vi "ExampleInstrument.AppLauncher.vi"() -> ()   [LabVIEW 2016, in "ExampleInstrument.lvclass"]
uses:
  ExampleInstrument.lvclass
  <vilib>/JKI/JKI SMO/SMO/Typedefs/SMOState --Enum.ctl
  Example Instrument UI/ExampleInstrument.UI.lvclass
  C:/Program Files (x86)/National Instruments/LabVIEW 2016/vi.lib/JKI/JKI SMO/SMO/SMO.lvclass
  C:/Program Files (x86)/National Instruments/LabVIEW 2016/vi.lib/JKI/JKI SMO/SMO.UI/SMO.UI.lvclass
  C:/Program Files (x86)/National Instruments/LabVIEW 2016/user.lib/LevyLab/Levylab Instruments/SMOs/Instrument/Instrument.lvclass
  <vilib>/JKI/JKI SMO/SMO/SMO.lvclass
  <vilib>/JKI/JKI SMO/SMO.UI/SMO.UI.lvclass
panel:
  out "error out":errorcluster
  in  "Splash Status":string="Push Start to Start..." caption="String"
  in  "Start":bool=TRUE
  in  "Stop":bool=TRUE
  out "UI SMO State":T1=enum."Stopped"
  out "SMO State":T1
  # "Example Instrument SMO Test Launcher"
  # "For instructions on how to use the JKI State Machine Objects, examples and video tutorials, visit:\nhttp://jki.net/state-machine-objects/\n\nJKI State Machine Objects™\nhttp://jki.net/state-machine-objects/\nCopyright (C) 2005-2015, JKI <info@jki.net>\nALL RIGHTS RESERVED"
  # "Starting Example Instrument..."
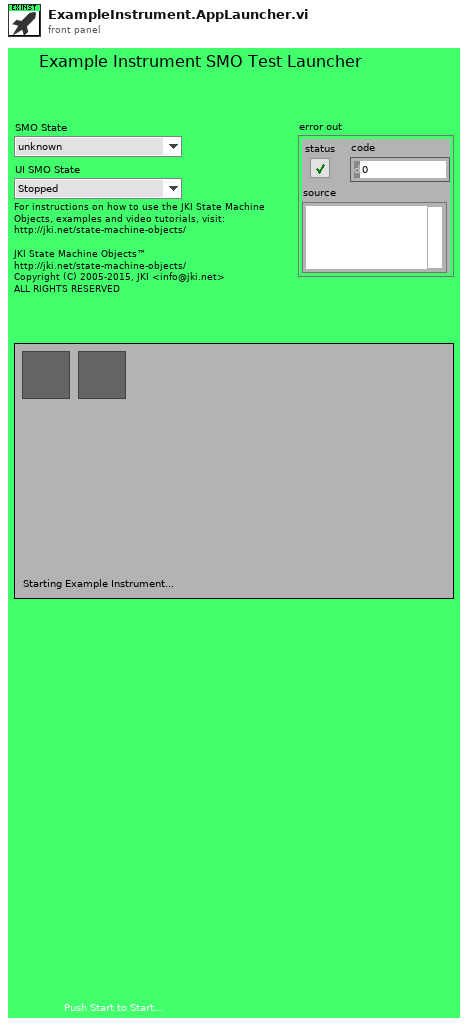
[diagram p1: front panel]
types:
  T1 = typedef "SMO.lvclass/SMOState --Enum.ctl" = enum16{"unknown", "Created", "Started", "Stopped"}
  T2 = enum32{"Invalid", "Standard", "Closed", "Hidden", "Minimized", "Maximized"}
  T3 = enum32{"invalid app kind", "Development System", "Run Time System", "Student Edition", "Embedded LabVIEW", "Evaluation", "Custom"}
  T4 = cluster{"Core":cluster{"Current VI Reference":refnum<vi>, "Close Panel on Exit?":bool}, "Instrument":refnum<class "ExampleInstrument.lvclass">, "Instrument UI":refnum<class "ExampleInstrument.UI.lvclass">}
  T5 = cluster{"Current VI Reference":refnum<vi>, "Close Panel on Exit?":bool}
  T6 = typedef "SMO.lvclass/Public Events.ctl" = cluster{"Error":refnum<user-event>, "State":refnum<user-event>, "Reserve State":refnum<user-event>}
  T7 = cluster{"Event Registration Refnum":refnum<event-registration>, "Event Registration Refnum":refnum<event-registration>}
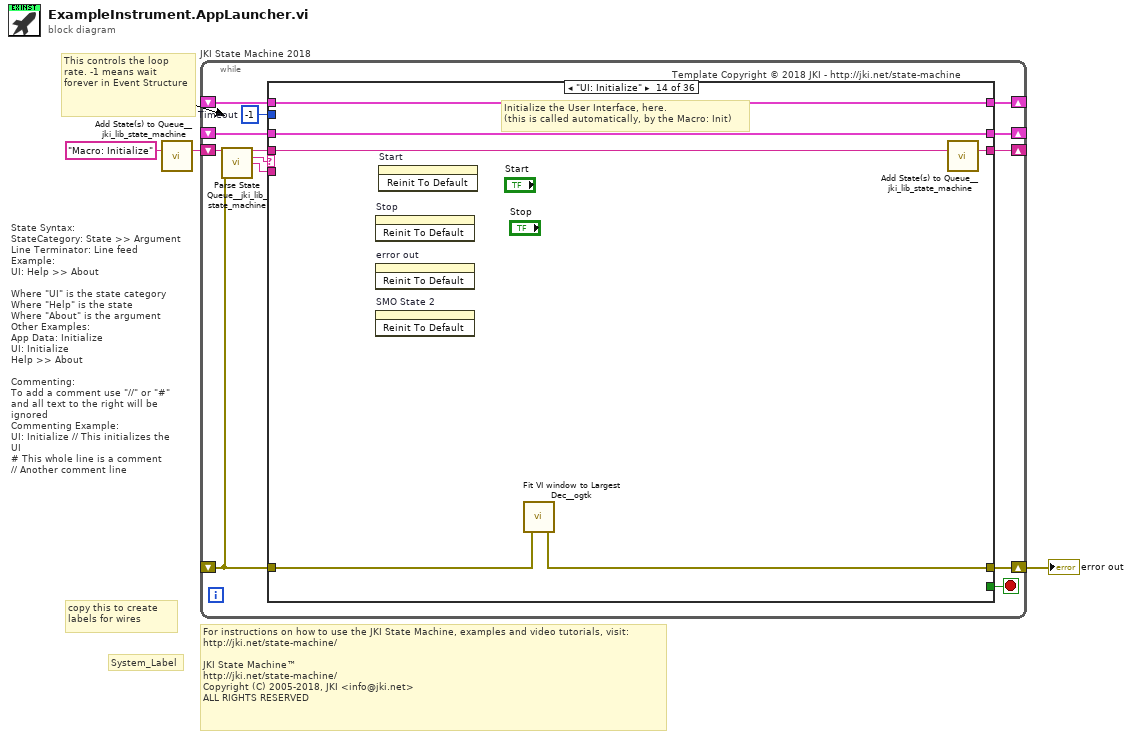
[diagram p0: block diagram]
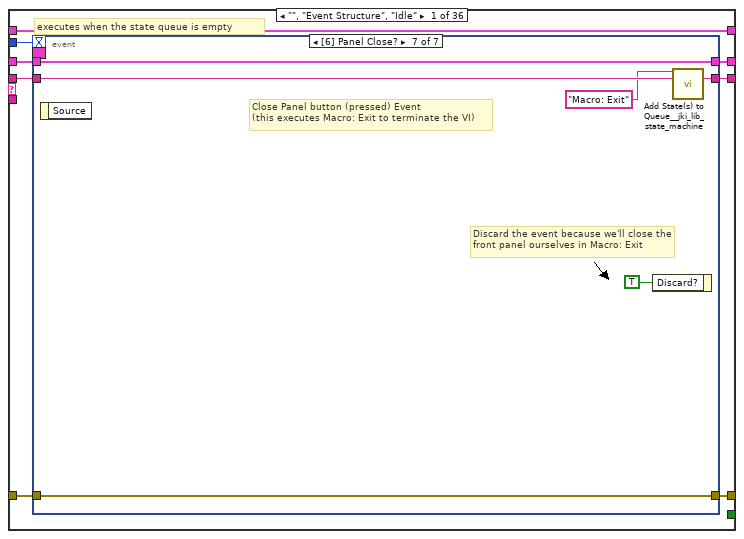
[diagram p2: hidden frame]
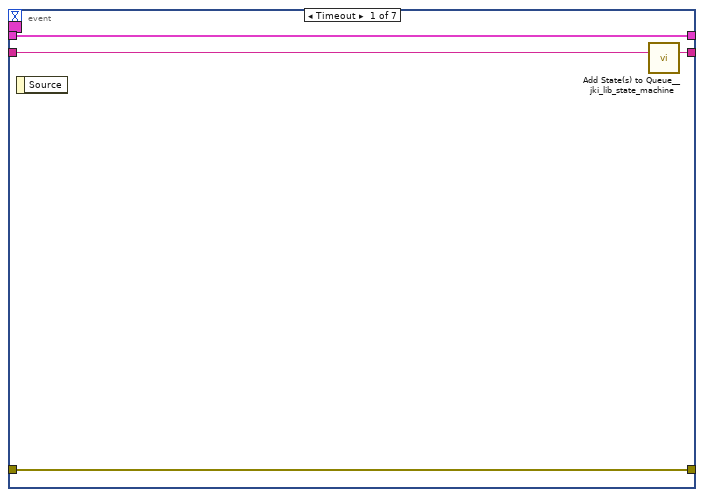
[diagram p3: hidden frame]
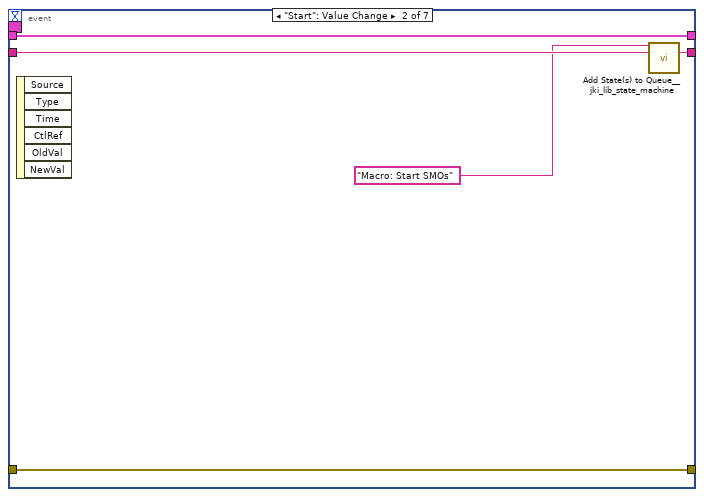
[diagram p4: hidden frame]
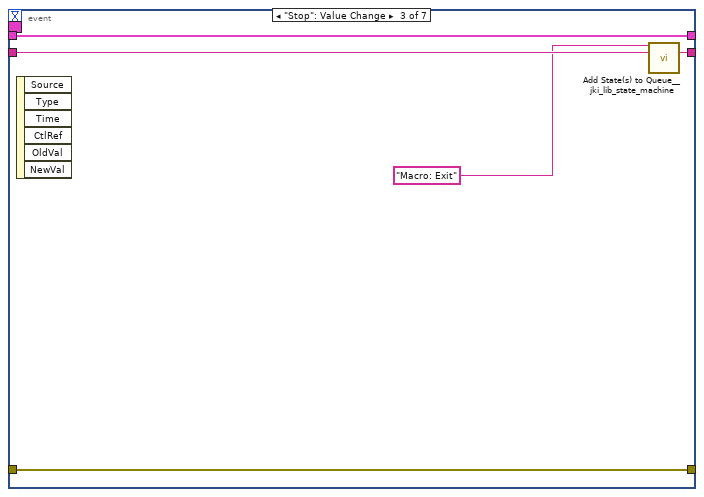
[diagram p5: hidden frame]
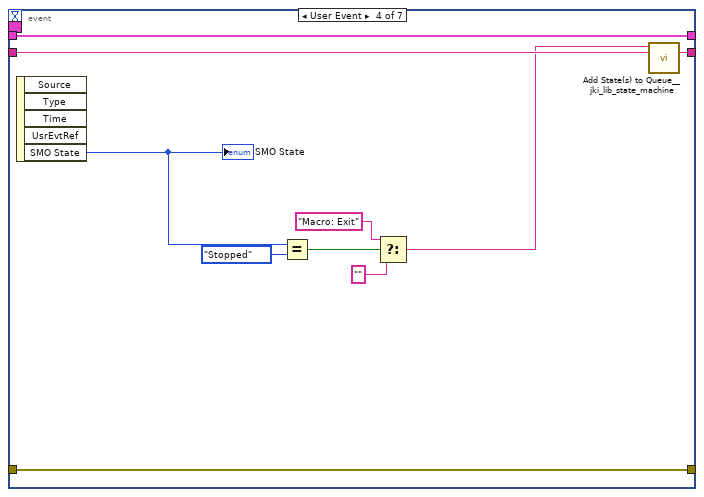
[diagram p6: hidden frame]
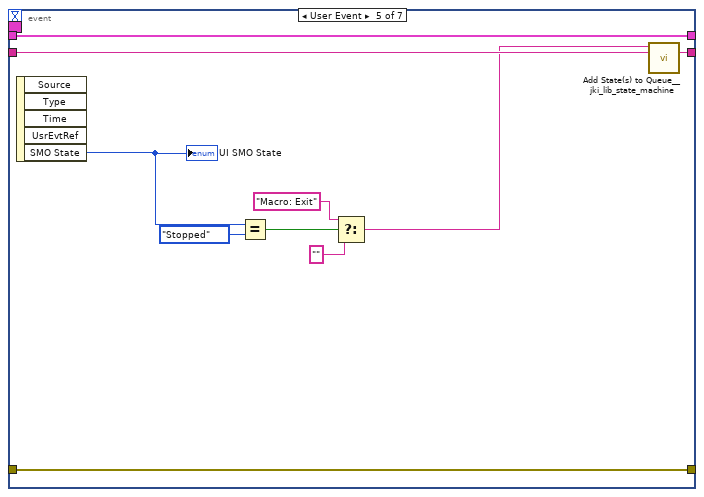
[diagram p7: hidden frame]
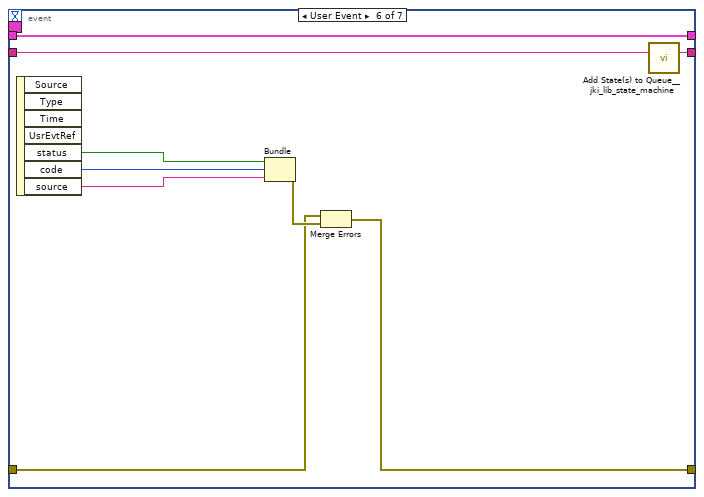
[diagram p8: hidden frame]
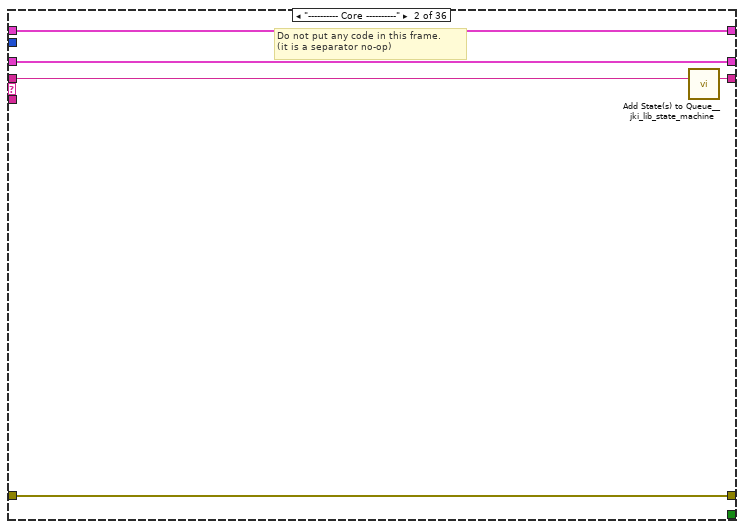
[diagram p9: hidden frame]
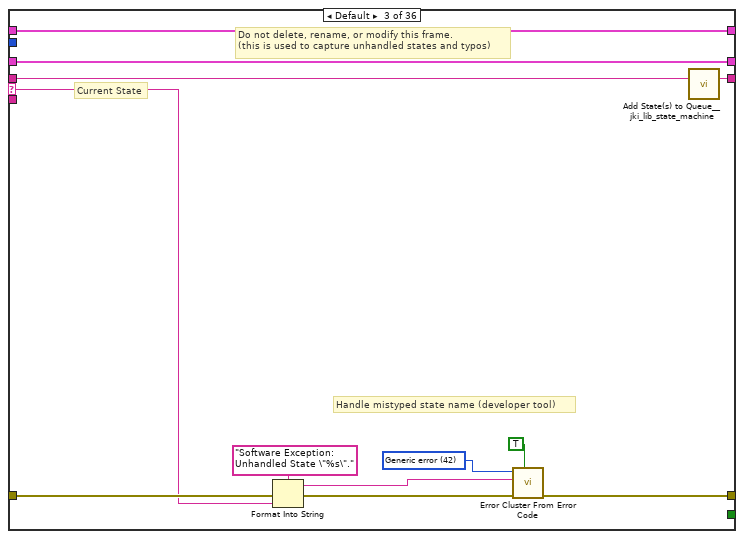
[diagram p10: hidden frame]
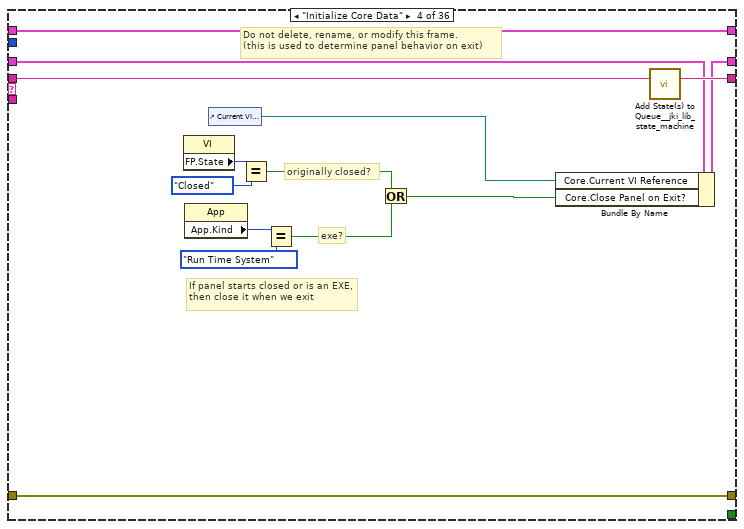
[diagram p11: hidden frame]
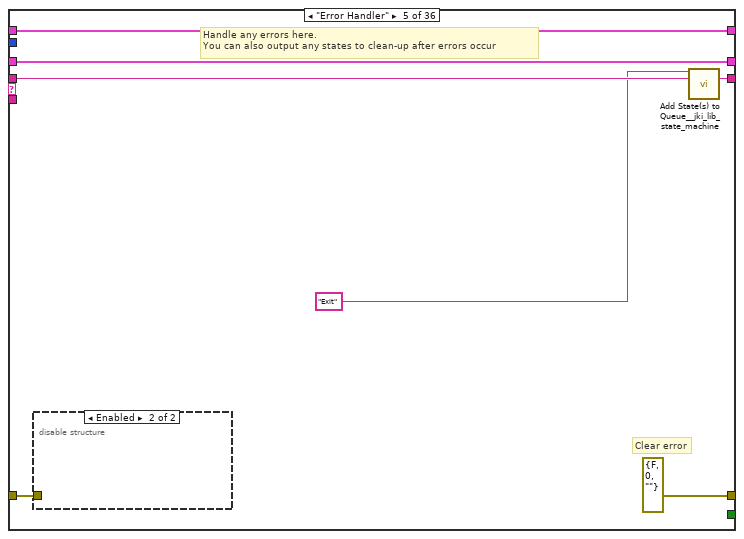
[diagram p12: hidden frame]
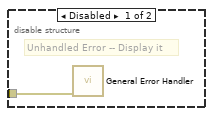
[diagram p13: hidden frame]
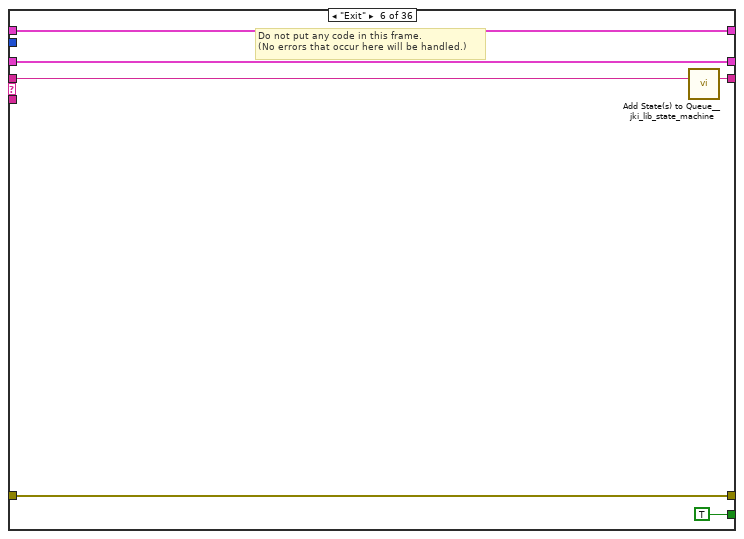
[diagram p14: hidden frame]
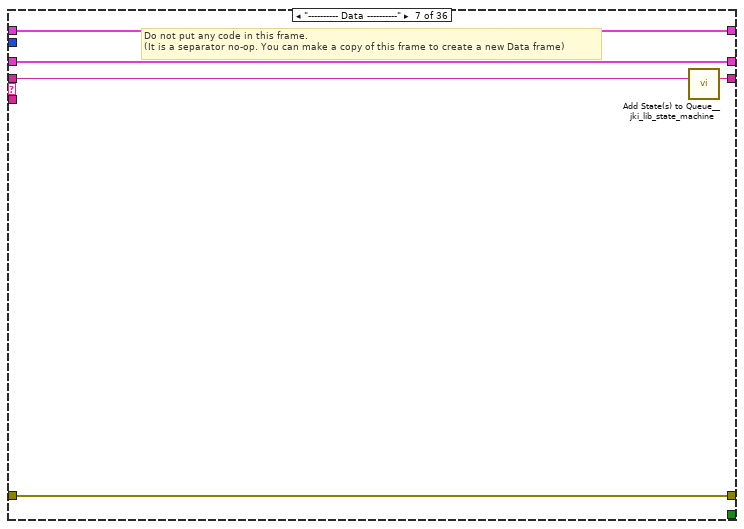
[diagram p15: hidden frame]
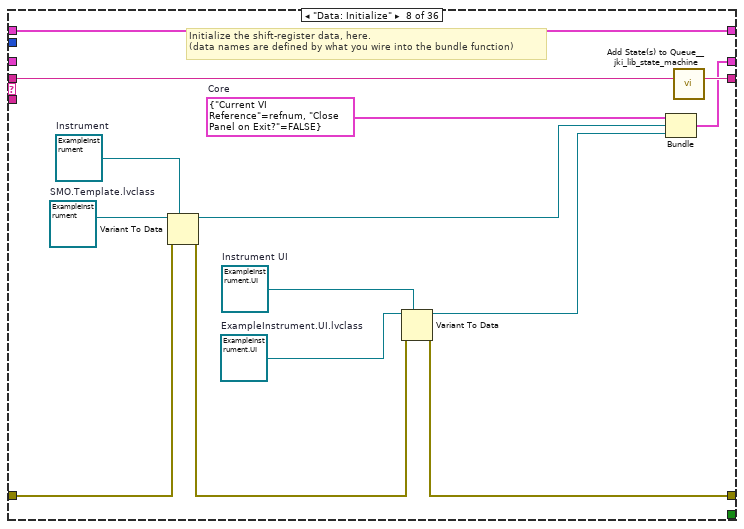
[diagram p16: hidden frame]
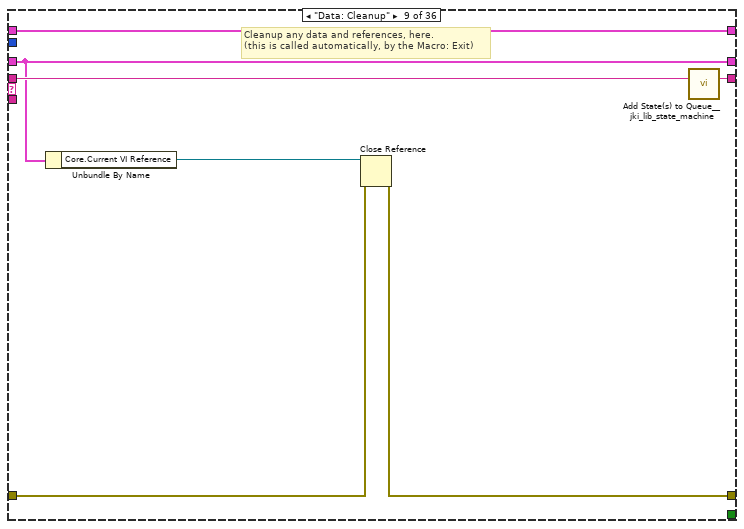
[diagram p17: hidden frame]
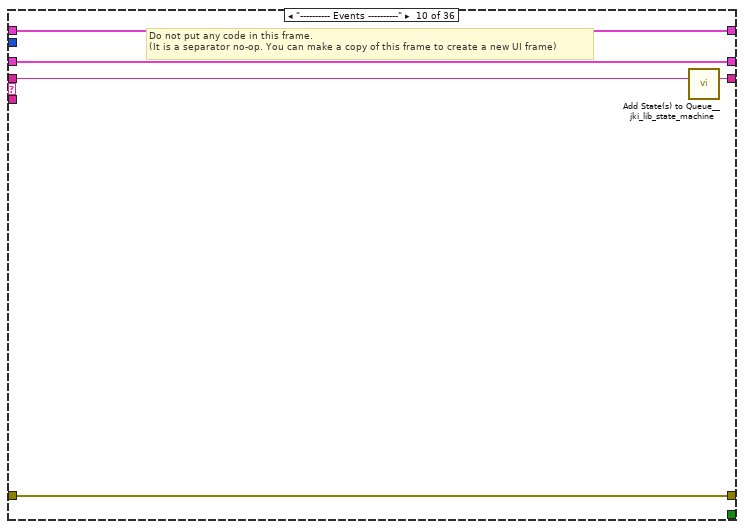
[diagram p18: hidden frame]
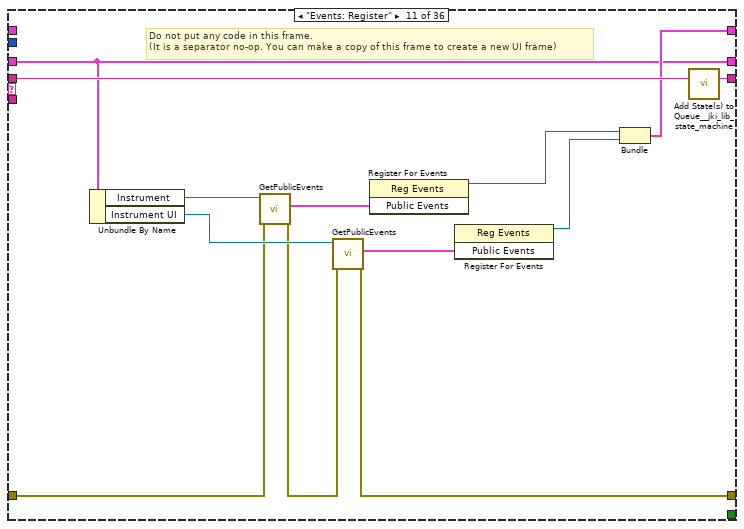
[diagram p19: hidden frame]
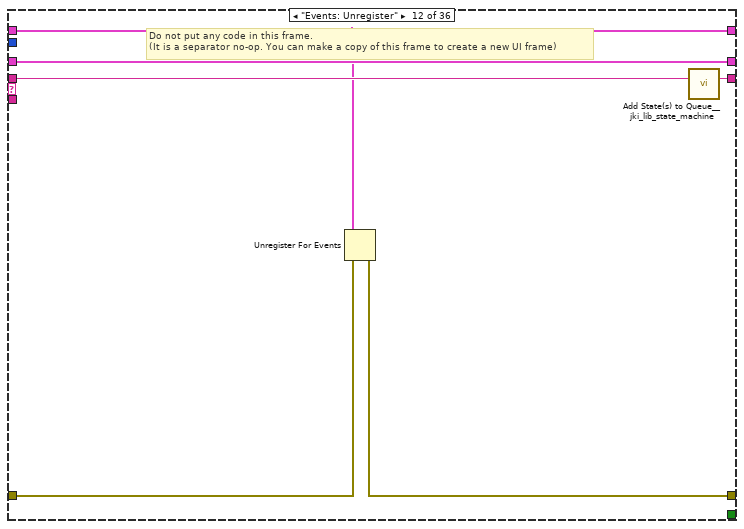
[diagram p20: hidden frame]
diagram:
  # "For instructions on how to use the JKI State Machine, examples and video tutorials, visit:\nhttp://jki.net/state-machine/\n\nJKI State Machine™\nhttp://jki.net/state-machine/\nCopyright (C) 2005-2018, JKI <info@jki.net>\nALL RIGHTS RESERVED"
  # "State Syntax:\nStateCategory: State >> Argument\nLine Terminator: Line feed\nExample:\nUI: Help >> About\n\nWhere \"UI\" is the state category\nWhere \"Help\" is the state\nWhere \"About\" is the argument\nOther Examples:\nApp Data: Initialize\nUI: Initialize\nHelp >> About\n\nCommenting:\nTo add a comment use \"//\" or \"#\" and all text to the right will be ignored\nCommenting Example:\nUI: Initialize // This initializes the UI\n# This whole line is a comment\n// Another comment line"
  # "copy this to create labels for wires"
  # "This controls the loop rate. -1 means wait forever in Event Structure"
  # "System_Label"
  n1 = call <vilib>:"Add State(s) to Queue__jki_lib_state_machine.vi"("State(s) in (\"\")"="Macro: Initialize") -> ("States Out"=w3:string)  [unwired: 14 in]
  n2 = while "JKI State Machine 2018" {
    shift-right: [w9] -> _
    shift-left: _ -> [w4]
    shift-right: [w12] -> w1
    shift-left: _ -> [w7]
    shift-right: [w11] -> _
    shift-left: w3 -> [w13]
    shift-right: [w6] -> _
    shift-left: _ -> [w5]
    stop <- w10 stop-if-true
    w8 = -1  # Timeout
    # "Template Copyright © 2018 JKI - http://jki.net/state-machine"
    n3 = call <vilib>:"Parse State Queue__jki_lib_state_machine.vi"("State Queue"=w13, "Error In (no error)"=w7) -> ("Remaining States"=w15:string, "Current State"=w16:string, "Arguments"=w14:string)  [unwired: 11 in]
    n4 = case shown="\"UI: Initialize\"" w16 {
      selector: w16 -> [_ _ w80 _ _ _ _ _ _ _ _ _ _ _ _ _ _ _ _ _ _ _ _ _ _ _ _ _ _ _ _ _ _ _ _ _]
      tunnel: w15 -> [w24 w78 w84 w104 w111 w118 w123 w137 w144 w149 w162 w168 w173 w179 w186 w198 w276 w281 w286 w292 w298 w304 w316 w321 w330 w339 w349 w356 w367 w382 w397 w412 w427 w436 w443 w448]
      tunnel: w14 -> [_ _ _ _ _ _ _ _ _ _ _ _ _ _ w181 w192 _ _ _ _ _ _ _ _ _ _ _ _ _ _ _ _ _ _ w440 _]
      tunnel: [w21 w76 w86 w101 errorcluster {"status"=FALSE, "code"=0, "source"=""} ("error out") w115 w121 w125 w140 w147 w151 w163 w171 w174 w182 w195 w266 w279 w284 w290 w296 w302 w314 w319 w326 w331 w340 w350 w363 w378 w393 w409 w424 w434 w438 w446] -> w12
      tunnel: w7 -> [w20 w76 w85 w101 w107 w115 w121 w127 w141 w147 w153 w164 w171 w176 w183 w196 w267 w279 w284 w290 w296 w302 w314 w319 w327 w332 w341 w351 w360 w374 w390 w407 w420 w434 w439 w446]
      tunnel: [w23 w77 w83 w103 w110 w117 w122 w136 w143 w148 w161 w167 w172 w178 w185 w197 w275 w280 w285 w291 w297 w303 w315 w320 w329 w338 w348 w355 w366 w381 w396 w411 w426 w435 w442 w447] -> w11
      tunnel: [_ _ _ _ _ TRUE _ _ _ _ _ _ _ _ _ _ _ _ _ _ _ _ _ _ _ _ _ _ _ _ _ _ _ _ _ _] -> w10
      tunnel: [w19 w75 w82 w102 w108 w116 w120 w135 w139 w146 w156 w166 w170 w177 w184 w194 w264 w278 w283 w289 w295 w301 w313 w318 w325 w334 w345 w353 w364 w379 w394 w408 w423 w433 w441 w445] -> w9
      tunnel: w8 -> [w18 _ _ _ _ _ _ _ _ _ _ _ _ _ _ _ _ _ _ _ _ _ _ _ _ _ _ _ _ _ _ _ _ _ _ _]
      tunnel: [w17 w74 w79 w91 w105 w113 w119 w133 w138 w145 w159 w165 w169 w175 w180 w191 w265 w277 w282 w287 w294 w300 w307 w317 w328 w337 w347 w354 w365 w380 w395 w410 w425 w432 w437 w444] -> w6
      tunnel: w5 -> [w17 w74 w79 w91 w105 w113 w119 w133 w138 w145 _ w165 w169 w175 w180 w191 w265 w277 w282 w287 w294 w300 w307 w317 w328 w337 w347 w354 w365 w380 w395 w410 w425 w432 w437 w444]
      tunnel: w4 -> [w22 w75 w82 w97 w108 w116 w120 _ w139 w146 w156 w166 w170 w177 w184 w194 w264 w278 w283 w289 w295 w301 w313 w318 w323 w335 w346 w353 w364 w379 w394 w408 w423 w433 w441 w445]
      frame "", "Event Structure", "Idle" {
        # "executes when the state queue is empty"
        n5 = event shown="[6] Panel Close?" {
          selector: w17 -> [_ _ _ _ _ _ _]
          dyn-events: _ -> [_ _ _ _ _ _ _]
          timeout: w18 -> [_ _ _ _ _ _ _]
          tunnel: w24 -> [w28 w33 w38 w48 w58 w67 w73]
          tunnel: [w27 w32 w37 w47 w57 w66 w72] -> w23
          tunnel: w22 -> [w25 w30 w35 w45 w55 w65 w70]
          tunnel: [w26 w31 w36 w46 w56 w62 w71] -> w21
          tunnel: w20 -> [w26 w31 w36 w46 w56 w63 w71]
          tunnel: [w25 w30 w35 w45 w55 w65 w70] -> w19
          event Timeout {
            n6 = event-data() -> ()  [unwired: 1 in, 1 out]
            n7 = call <vilib>:"Add State(s) to Queue__jki_lib_state_machine.vi"("State(s) in (\"\")"=w28) -> ("States Out"=w27:string)  [unwired: 14 in]
          }
          event "Start": Value Change {
            n8 = event-data() -> ()  [unwired: 1 in, 6 out]
            n9 = call <vilib>:"Add State(s) to Queue__jki_lib_state_machine.vi"("State(s) in Front (\"\")"="Macro: Start SMOs" ("State(s) in Front (\"\")"), "State(s) in (\"\")"=w33) -> ("States Out"=w32:string)  [unwired: 13 in]
          }
          event "Stop": Value Change {
            n10 = event-data() -> ()  [unwired: 1 in, 6 out]
            n11 = call <vilib>:"Add State(s) to Queue__jki_lib_state_machine.vi"("State(s) in Front (\"\")"="Macro: Exit" ("State(s) in Front (\"\")"), "State(s) in (\"\")"=w38) -> ("States Out"=w37:string)  [unwired: 13 in]
          }
          event User Event {
            n12 = event-data() -> ("SMO State"=w40:T1)  [unwired: 1 in, 4 out]
            "SMO State" <- w40
            n13 = Equal?(x=w40, y=SMOState_--Enum."Stopped") -> (x = y?=w43:bool)
            n14 = Select(t="Macro: Exit", s=w43, f="" ("State(s) in Front (\"\")")) -> (s? t:f=w39:string)
            n15 = call <vilib>:"Add State(s) to Queue__jki_lib_state_machine.vi"("State(s) in Front (\"\")"=w39, "State(s) in (\"\")"=w48) -> ("States Out"=w47:string)  [unwired: 13 in]
          }
          event User Event {
            n16 = event-data() -> ("SMO State"=w49:T1)  [unwired: 1 in, 4 out]
            "UI SMO State" <- w49
            n17 = Equal?(x=w49, y=SMOState_--Enum."Stopped") -> (x = y?=w53:bool)
            n18 = Select(t="Macro: Exit", s=w53, f="" ("State(s) in Front (\"\")")) -> (s? t:f=w51:string)
            n19 = call <vilib>:"Add State(s) to Queue__jki_lib_state_machine.vi"("State(s) in Front (\"\")"=w51, "State(s) in (\"\")"=w58) -> ("States Out"=w57:string)  [unwired: 13 in]
          }
          event User Event {
            n20 = event-data() -> ("status"=w59:bool, "code"=w61:i32, "source"=w60:string)  [unwired: 1 in, 4 out]
            n21 = Bundle("status"=w59, "code"=w61, "source"=w60) -> (w64:errorcluster)  [unwired: 1 in]
            n22 = Merge Errors(w63, w64) -> (w62:errorcluster)
            n23 = call <vilib>:"Add State(s) to Queue__jki_lib_state_machine.vi"("State(s) in (\"\")"=w67) -> ("States Out"=w66:string)  [unwired: 14 in]
          }
          event Panel Close? {
            # "Discard the event because we'll close the front panel ourselves in Macro: Exit"
            # "Close Panel button (pressed) Event\n(this executes Macro: Exit to terminate the VI)"
            n24 = event-data() -> ()  [unwired: 1 in, 1 out]
            n25 = event-data("Discard?"=TRUE) -> ()  [unwired: 1 in, 1 out]
            n26 = call <vilib>:"Add State(s) to Queue__jki_lib_state_machine.vi"("State(s) in Front (\"\")"="Macro: Exit", "State(s) in (\"\")"=w73) -> ("States Out"=w72:string)  [unwired: 13 in]
          }
        }
      }
      frame "---------- Core ----------" {
        # "Do not put any code in this frame.\n(it is a separator no-op)"
        n27 = call <vilib>:"Add State(s) to Queue__jki_lib_state_machine.vi"("State(s) in (\"\")"=w78) -> ("States Out"=w77:string)  [unwired: 14 in]
      }
      frame Default {
        w89 = 42 items=["No error", "Argument error", "Memory is full", "Out of zone", "End of file", "File already open", "Generic file I/O error", "File not found", "File permission error", "Disk is full", "Duplicate path", "Too many files open", "System feature not enabled", "Resource file not found", "Cannot add resource", "Resource not found", "Image not found", "Image memory error", "Pen does not exist", "Config type invalid", "Config token not found", "Config parse error", "Config memory error", "Bad external code format", "Bad external code offset", "External code not present", "Null window", "Destroy window error", "Null menu", "Print aborted", "Bad print record", "Print driver error", "Windows error during printing", "Memory error during printing", "Print dialog error", "Generic print error", "Invalid device refnum", "Device not found", "Device parameter error", "Device unit error", "Cannot open device", "Device call aborted", "Generic error", "Cancelled by user", "Object ID too low", "Object ID too high", "Object not in heap", "Unknown heap", "Unknown object (invalid DefProc)", "Unknown object (DefProc not in table)", "Message out of range", "Invalid (null) method", "Unknown message", "Manager call not supported", "Bad address", "Network operation in progress", "Network operation timed out", "Connection is busy", "Network attribute not supported", "Network error", "Address in use", "System out of memory", "Connection aborted", "Connection refused", "Not connected", "Already connected", "Connection closed", "Initialization error (interapplication manager)", "Bad occurrence", "Wait on unbound occurrence handler", "Occurrence queue overflow", "Datalog type conflict", "Unused", "Unrecognized type (interapplication manager)", "Memory corrupt", "Failed to make temporary DLL", "Old CIN version", "Drag socket not found", "Failed to load drop-object", "Failed to register OLE object", "Failed to release OLE object", "Format specifier type mismatch", "Unknown format specifier", "Too few format specifiers", "Too many format specifiers", "Scan failed", "Newer CIN version", "Error converting to variant", "Runtime menu error", "Password tampered", "Variant attribute not found", "Incompatible variant data type", "Event data is not available", "Event Store is not present", "Occurrence is not found", "Event Queue is not created", "Event info is not available", "Refnum passed is NULL", "Error retrieving Class GUID", "Error retrieving CoClass GUID", "Error retrieving TypeLib GUID.", "Bad built application magic bytes.", "Specific driver is different from the specific driver associated with the Logical Name.", "There is no session opened to the class driver.", "Max Error", "MAX - Error with config objects", "MAX - Error loading configuration", "MAX - Group not supported"]
        # "Current State"
        # "Do not delete, rename, or modify this frame.\n(this is used to capture unhandled states and typos)"
        # "Handle mistyped state name (developer tool)"
        n28 = Format Into String(format string="Software Exception: Unhandled State \"%s\"." ("message"), error in=w85, w80) -> (resulting string=w88:string, error out=w87:errorcluster)  [unwired: 1 in]
        n29 = call <vilib>:"Error Cluster From Error Code.vi"("show call chain? (False)"=TRUE, "error in (no error)"=w87, "error message (\"\")"=w88, "error code (0)"=w89) -> ("error out"=w86:errorcluster)  [unwired: 5 in]
        n30 = call <vilib>:"Add State(s) to Queue__jki_lib_state_machine.vi"("State(s) in (\"\")"=w84) -> ("States Out"=w83:string)  [unwired: 14 in]
      }
      frame "Initialize Core Data" {
        # "Do not delete, rename, or modify this frame.\n(this is used to determine panel behavior on exit)"
        # "originally closed?"
        # "exe?"
        # "If panel starts closed or is an EXE, then close it when we exit"
        n31 = property class="VI"() -> ("FP.State"=w94:T2)  [unwired: 2 in, 2 out]
        n32 = property class="App"() -> ("App.Kind"=w100:T3)  [unwired: 2 in, 2 out]
        n33 = control-ref of="Current VI Reference"() -> (w95:refnum<vi>)
        n34 = Equal?(x=w94, y=T2."Closed" ("Front Panel Window:State")) -> (x = y?=w92:bool)
        n35 = Equal?(x=w100, y=T3."Run Time System" ("Application:Kind")) -> (x = y?=w98:bool)
        n36 = Or(x=w92, y=w98) -> (x .or. y?=w96:bool)
        n37 = Bundle By Name(cluster=w97, "Core.Current VI Reference"=w95, "Core.Close Panel on Exit?"=w96) -> (w102:T4)
        n38 = call <vilib>:"Add State(s) to Queue__jki_lib_state_machine.vi"("State(s) in (\"\")"=w104) -> ("States Out"=w103:string)  [unwired: 14 in]
      }
      frame "Error Handler" {
        # "Handle any errors here.\nYou can also output any states to clean-up after errors occur"
        # "Clear error"
        n39 = disable-structure shown="Enabled" {
          disable-tunnel: w107 -> [w112 _]
          frame Disabled {
            # "Unhandled Error -- Display it"
            n40 = call <vilib>:"General Error Handler.vi"("error in (no error)"=w112) -> ()  [unwired: 10 in, 5 out]
          }
          frame Enabled {
          }
        }
        n41 = call <vilib>:"Add State(s) to Queue__jki_lib_state_machine.vi"("State(s) in Front (\"\")"="Exit", "State(s) in (\"\")"=w111) -> ("States Out"=w110:string)  [unwired: 13 in]
      }
      frame "Exit" {
        # "Do not put any code in this frame.\n(No errors that occur here will be handled.)"
        n42 = call <vilib>:"Add State(s) to Queue__jki_lib_state_machine.vi"("State(s) in (\"\")"=w118) -> ("States Out"=w117:string)  [unwired: 14 in]
      }
      frame "---------- Data ----------" {
        # "Do not put any code in this frame.\n(It is a separator no-op. You can make a copy of this frame to create a new Data frame)"
        n43 = call <vilib>:"Add State(s) to Queue__jki_lib_state_machine.vi"("State(s) in (\"\")"=w123) -> ("States Out"=w122:string)  [unwired: 14 in]
      }
      frame "Data: Initialize" {
        w129 = refnum<class "ExampleInstrument.UI.lvclass"> refnum  # Instrument UI
        w131 = refnum<class "ExampleInstrument.lvclass"> refnum  # Instrument
        w132 = refnum<class "ExampleInstrument.lvclass"> refnum  # SMO.Template.lvclass
        w124 = refnum<class "ExampleInstrument.UI.lvclass"> refnum  # ExampleInstrument.UI.lvclass
        w134 = T5 {"Current VI Reference"=refnum, "Close Panel on Exit?"=FALSE}  # Core
        # "Initialize the shift-register data, here.\n(data names are defined by what you wire into the bundle function)"
        n44 = Variant To Data(error in=w127, type=w131, Variant=w132) -> (data=w130:refnum<class "ExampleInstrument.lvclass">, error out=w126:errorcluster)
        n45 = Variant To Data(error in=w126, type=w129, Variant=w124) -> (data=w128:refnum<class "ExampleInstrument.UI.lvclass">, error out=w125:errorcluster)
        n46 = Bundle("Core"=w134, "Instrument"=w130, "Instrument UI"=w128) -> (w135:T4)  [unwired: 1 in]
        n47 = call <vilib>:"Add State(s) to Queue__jki_lib_state_machine.vi"("State(s) in (\"\")"=w137) -> ("States Out"=w136:string)  [unwired: 14 in]
      }
      frame "Data: Cleanup" {
        # "Cleanup any data and references, here.\n(this is called automatically, by the Macro: Exit)"
        n48 = Unbundle By Name(w139) -> ("Core.Current VI Reference"=w142:refnum<vi>)
        n49 = Close Reference(reference=w142, error in (no error)=w141) -> (error out=w140:errorcluster)
        n50 = call <vilib>:"Add State(s) to Queue__jki_lib_state_machine.vi"("State(s) in (\"\")"=w144) -> ("States Out"=w143:string)  [unwired: 14 in]
      }
      frame "---------- Events ----------" {
        # "Do not put any code in this frame.\n(It is a separator no-op. You can make a copy of this frame to create a new UI frame)"
        n51 = call <vilib>:"Add State(s) to Queue__jki_lib_state_machine.vi"("State(s) in (\"\")"=w149) -> ("States Out"=w148:string)  [unwired: 14 in]
      }
      frame "Events: Register" {
        # "Do not put any code in this frame.\n(It is a separator no-op. You can make a copy of this frame to create a new UI frame)"
        n52 = Unbundle By Name(w156) -> ("Instrument"=w155:refnum<class "ExampleInstrument.lvclass">, "Instrument UI"=w154:refnum<class "ExampleInstrument.UI.lvclass">)
        n53 = call <vilib>:"GetPublicEvents.vi"("error in (no error)"=w153, "SMO"=w155) -> ("error out"=w152:errorcluster, "Public Events"=w157:T6)  [unwired: 7 in, 1 out]
        n54 = call <vilib>:"GetPublicEvents.vi"("error in (no error)"=w152, "SMO"=w154) -> ("error out"=w151:errorcluster, "Public Events"=w158:T6)  [unwired: 7 in, 1 out]
        n55 = register-events(w157) -> (reference out=w160:refnum<event-registration>)  [unwired: 2 in, 1 out]
        n56 = register-events(w158) -> (reference out=w150:refnum<event-registration>)  [unwired: 2 in, 1 out]
        n57 = Bundle("Event Registration Refnum"=w160, "Event Registration Refnum"=w150) -> (w159:T7)  [unwired: 1 in]
        n58 = call <vilib>:"Add State(s) to Queue__jki_lib_state_machine.vi"("State(s) in (\"\")"=w162) -> ("States Out"=w161:string)  [unwired: 14 in]
      }
      frame "Events: Unregister" {
        # "Do not put any code in this frame.\n(It is a separator no-op. You can make a copy of this frame to create a new UI frame)"
        n59 = Unregister For Events(event registration refnum=w165, error in=w164) -> (error out=w163:errorcluster)
        n60 = call <vilib>:"Add State(s) to Queue__jki_lib_state_machine.vi"("State(s) in (\"\")"=w168) -> ("States Out"=w167:string)  [unwired: 14 in]
      }
      frame "---------- UI ----------" {
        # "Do not put any code in this frame.\n(It is a separator no-op. You can make a copy of this frame to create a new UI frame)"
        n61 = call <vilib>:"Add State(s) to Queue__jki_lib_state_machine.vi"("State(s) in (\"\")"=w173) -> ("States Out"=w172:string)  [unwired: 14 in]
      }
      frame "UI: Initialize" {
        # "Initialize the User Interface, here.\n(this is called automatically, by the Macro: Init)"
        n62 = invoke on="Stop" class="Bool (strict)" method="Reinit To Default"() -> ()  [unwired: 3 in, 3 out]
        n63 = invoke on="error out" class="Clust (strict)" method="Reinit To Default"() -> ()  [unwired: 3 in, 3 out]
        n64 = invoke on="SMO State 2" class="Enum (strict)" method="Reinit To Default"() -> ()  [unwired: 3 in, 3 out]
        n65 = invoke on="Start" class="Bool (strict)" method="Reinit To Default"() -> ()  [unwired: 3 in, 3 out]
        n66 = call <userlib>:"Fit VI window to Largest Dec__ogtk.vi"("error in (no error)"=w176) -> ("error out"=w174:errorcluster)  [unwired: 5 in, 1 out]
        n67 = call <vilib>:"Add State(s) to Queue__jki_lib_state_machine.vi"("State(s) in (\"\")"=w179) -> ("States Out"=w178:string)  [unwired: 14 in]
      }
      frame "UI: Cursor Set" {
        # "Argument"
        # "Set and Unset Cursor Busy.\n(Usage: \"UI: Cursor Set >> Busy|Idle\")"
        n68 = case shown="\"Idle\", Default" w181 {
          tunnel: w183 -> [w188 w190]
          tunnel: [w187 w189] -> w182
          frame "Idle", Default {
            n69 = call <vilib>:"Unset Busy.vi"("error in (no error)"=w188) -> ("error out"=w187:errorcluster)  [unwired: 10 in]
          }
          frame "Busy" {
            n70 = call <vilib>:"Set Busy.vi"("error in (no error)"=w190) -> ("error out"=w189:errorcluster)  [unwired: 9 in, 1 out]
          }
        }
        n71 = call <vilib>:"Add State(s) to Queue__jki_lib_state_machine.vi"("State(s) in (\"\")"=w186) -> ("States Out"=w185:string)  [unwired: 14 in]
      }
      frame "UI: Front Panel State" {
        # "Argument"
        # "Set Front Panel Open or Closed\n(Usage: \"UI: Front Panel State >> Open|Close\")"
        n72 = Unbundle By Name(w194) -> ("Core.Current VI Reference"=w193:refnum<vi>)
        n73 = case shown="\"Maximize\", \"Maximized\"" w192 {
          tunnel: w196 -> [w204 w219 w230 w243 w256]
          tunnel: [w206 w220 w232 w245 w258] -> w195
          tunnel: w193 -> [w205 w217 w231 w244 w257]
          frame "Open", "Standard", Default {
            w199 = T2."Standard" ("State")
            n74 = property class="VI"(reference=w205, error in=w204) -> (reference out=w202:refnum<vi>, error out=w203:errorcluster, "FP.State"=w201:T2)
            n75 = Not Equal?(x=w201, y=w199) -> (x != y?=w200:bool)
            n76 = case shown="True" w200 {
              tunnel: [w210 w212] -> w206
              tunnel: w203 -> [w209 w212]
              tunnel: w202 -> [w208 _]
              tunnel: w199 -> [w207 _]
              frame True {
                n77 = invoke class="VI" method="FP.Open"(reference=w208, error in=w209, "Activate"=TRUE, "State"=w207) -> (error out=w210:errorcluster)  [unwired: 1 in, 4 out]
              }
              frame False {
              }
            }
          }
          frame "Close", "Closed" {
            n78 = property class="VI"(reference=w217, error in=w219) -> (reference out=w216:refnum<vi>, error out=w218:errorcluster, "FP.State"=w214:T2)
            n79 = Not Equal?(x=w214, y=T2."Closed" ("Front Panel Window:State")) -> (x != y?=w213:bool)
            n80 = case shown="True" w213 {
              tunnel: [w221 w224] -> w220
              tunnel: w218 -> [w221 w223]
              tunnel: w216 -> [_ w222]
              frame False {
              }
              frame True {
                n81 = invoke class="VI" method="FP.Close"(reference=w222, error in=w223) -> (error out=w224:errorcluster)  [unwired: 1 in, 2 out]
              }
            }
          }
          frame "Hidden", "Hide" {
            w225 = T2."Hidden" ("State")
            n82 = property class="VI"(reference=w231, error in=w230) -> (reference out=w228:refnum<vi>, error out=w229:errorcluster, "FP.State"=w227:T2)
            n83 = Not Equal?(x=w227, y=w225) -> (x != y?=w226:bool)
            n84 = case shown="True" w226 {
              tunnel: [w236 w237] -> w232
              tunnel: w229 -> [w235 w237]
              tunnel: w228 -> [w234 _]
              tunnel: w225 -> [w233 _]
              frame True {
                n85 = invoke class="VI" method="FP.Open"(reference=w234, error in=w235, "State"=w233) -> (error out=w236:errorcluster)  [unwired: 2 in, 4 out]
              }
              frame False {
              }
            }
          }
          frame "Minimize", "Minimized" {
            w238 = T2."Minimized" ("State")
            n86 = property class="VI"(reference=w244, error in=w243) -> (reference out=w241:refnum<vi>, error out=w242:errorcluster, "FP.State"=w240:T2)
            n87 = Not Equal?(x=w240, y=w238) -> (x != y?=w239:bool)
            n88 = case shown="True" w239 {
              tunnel: [w249 w250] -> w245
              tunnel: w242 -> [w248 w250]
              tunnel: w241 -> [w247 _]
              tunnel: w238 -> [w246 _]
              frame True {
                n89 = invoke class="VI" method="FP.Open"(reference=w247, error in=w248, "State"=w246) -> (error out=w249:errorcluster)  [unwired: 2 in, 4 out]
              }
              frame False {
              }
            }
          }
          frame "Maximize", "Maximized" {
            w251 = T2."Maximized" ("State")
            n90 = property class="VI"(reference=w257, error in=w256) -> (reference out=w254:refnum<vi>, error out=w255:errorcluster, "FP.State"=w253:T2)
            n91 = Not Equal?(x=w253, y=w251) -> (x != y?=w252:bool)
            n92 = case shown="True" w252 {
              tunnel: [w262 w263] -> w258
              tunnel: w255 -> [w261 w263]
              tunnel: w254 -> [w260 _]
              tunnel: w251 -> [w259 _]
              frame True {
                n93 = invoke class="VI" method="FP.Open"(reference=w260, error in=w261, "State"=w259) -> (error out=w262:errorcluster)  [unwired: 2 in, 4 out]
              }
              frame False {
              }
            }
          }
        }
        n94 = call <vilib>:"Add State(s) to Queue__jki_lib_state_machine.vi"("State(s) in (\"\")"=w198) -> ("States Out"=w197:string)  [unwired: 14 in]
      }
      frame "UI: Set Background Color" {
        # "Do not put any code in this frame.\n(It is a separator no-op. You can make a copy of this frame to create a new UI frame)"
        n95 = property class="VI"(error in=w267) -> (error out=w269:errorcluster, "Panel"=w270:refnum<vi>)  [unwired: 1 in, 1 out]
        n96 = property class="Pnl"(reference=w270, error in=w269) -> (error out=w268:errorcluster, "Panes[]"=w271:refnum<vi>[])  [unwired: 1 out]
        n97 = Index Array(array=w271, index=0) -> (element=w273:refnum<vi>)
        n98 = property class="Pane"(reference=w273, error in=w268, "PaneColor"=u32 16777238 ("Color Box")) -> (error out=w266:errorcluster)  [unwired: 1 out]
        n99 = call <vilib>:"Add State(s) to Queue__jki_lib_state_machine.vi"("State(s) in (\"\")"=w276) -> ("States Out"=w275:string)  [unwired: 14 in]
      }
      frame "UI: Exit" {
        # "Do not put any code in this frame.\n(It is a separator no-op. You can make a copy of this frame to create a new UI frame)"
        n100 = invoke on="Start" class="Bool (strict)" method="Reinit To Default"() -> ()  [unwired: 3 in, 3 out]
        n101 = invoke on="Stop" class="Bool (strict)" method="Reinit To Default"() -> ()  [unwired: 3 in, 3 out]
        n102 = call <vilib>:"Add State(s) to Queue__jki_lib_state_machine.vi"("State(s) in (\"\")"=w281) -> ("States Out"=w280:string)  [unwired: 14 in]
      }
      frame "---------- Macro ----------" {
        # "Do not put any code in this frame.\n(It is a separator no-op. You can make a copy of this frame to create a new Macro frame)"
        n103 = call <vilib>:"Add State(s) to Queue__jki_lib_state_machine.vi"("State(s) in (\"\")"=w286) -> ("States Out"=w285:string)  [unwired: 14 in]
      }
      frame "Macro: Initialize" {
        # "Initialization Macro\n(This is called once, when the VI starts)"
        n104 = call <vilib>:"Add State(s) to Queue__jki_lib_state_machine.vi"("State(s) in Front (\"\")"="Data: Initialize\nInitialize Core Data\n//Events: Register\nUI: Initialize\nUI: Front Panel State >> Open\nUI: Set Background Color\nSplash: Set Status >> Push Start to Start...", "State(s) in (\"\")"=w292) -> ("States Out"=w291:string)  [unwired: 13 in]
      }
      frame "Macro: Start SMOs" {
        # "Do not put any code in this frame.\n(It is a separator no-op. You can make a copy of this frame to create a new Macro frame)"
        n105 = call <vilib>:"Add State(s) to Queue__jki_lib_state_machine.vi"("State(s) in Front (\"\")"="Splash: Set Status >> Starting Instrument...\nSMO: Create Instrument\nSMO: Create Instrument UI\nEvents: Register\nSMO: Start Instrument\nSplash: Set Status >> Instrument Process Started...\nSplash: Set Status >> Starting User Interface...\nSMO: Start Instrument UI\nUI: Front Panel State >> Hide\nSMO: Show Instrument UI" ("State(s) in Front (\"\")"), "State(s) in (\"\")"=w298) -> ("States Out"=w297:string)  [unwired: 13 in]
      }
      frame "Macro: Stop SMOs" {
        # "Do not put any code in this frame.\n(It is a separator no-op. You can make a copy of this frame to create a new Macro frame)"
        n106 = call <vilib>:"Add State(s) to Queue__jki_lib_state_machine.vi"("State(s) in Front (\"\")"="SMO: Destroy Instrument\nSMO: Hide Instrument UI\nSMO: Stop Instrument UI\nSMO: Destroy Instrument UI" ("State(s) in Front (\"\")"), "State(s) in (\"\")"=w304) -> ("States Out"=w303:string)  [unwired: 13 in]
      }
      frame "Macro: Exit" {
        # "Exit Macro\n(This is called once, when the VI exits)"
        n107 = Unbundle By Name(w313) -> ("Core.Close Panel on Exit?"=w312:bool)
        n108 = Select(t="UI: Front Panel State >> Open", s=w312, f="") -> (s? t:f=w309:string)
        n109 = call <vilib>:"Add State(s) to Queue__jki_lib_state_machine.vi"("State(s) in Front (\"\")"="UI: Front Panel State >> Open\nUI: Exit", "State(s) in (\"\")"=w309, "State(s) at Back (\"\")"="Macro: Stop SMOs\nData: Cleanup\nEvents: Unregister\nExit") -> ("States Out"=w308:string)  [unwired: 12 in]
        n110 = call <vilib>:"Add State(s) to Queue__jki_lib_state_machine.vi"("State(s) in Front (\"\")"=w308, "State(s) in (\"\")"=w316) -> ("States Out"=w315:string)  [unwired: 13 in]
      }
      frame "---------- SMO ----------" {
        # "Do not put any code in this frame.\n(It is a separator no-op. You can make a copy of this frame to create a new Macro frame)"
        n111 = call <vilib>:"Add State(s) to Queue__jki_lib_state_machine.vi"("State(s) in (\"\")"=w321) -> ("States Out"=w320:string)  [unwired: 14 in]
      }
      frame "SMO: Create Instrument" {
        # "Do not put any code in this frame.\n(It is a separator no-op. You can make a copy of this frame to create a new Macro frame)"
        n112 = Unbundle By Name(w323) -> ("Instrument"=w322:refnum<class "ExampleInstrument.lvclass">)
        n113 = call-dynamic "Create Instrument.vi"("error in (no error)"=w327, "Instrument in"=w322) -> ("error out"=w326:errorcluster, "Instrument out"=w324:refnum<class "ExampleInstrument.lvclass">)  [unwired: 8 in]
        n114 = Bundle By Name(cluster=w323, "Instrument"=w324) -> (w325:T4)
        n115 = call <vilib>:"Add State(s) to Queue__jki_lib_state_machine.vi"("State(s) in (\"\")"=w330) -> ("States Out"=w329:string)  [unwired: 14 in]
      }
      frame "SMO: Start Instrument" {
        # "Do not put any code in this frame.\n(It is a separator no-op. You can make a copy of this frame to create a new Macro frame)"
        n116 = Unbundle By Name(w335) -> ("Instrument"=w336:refnum<class "ExampleInstrument.lvclass">)
        n117 = call <vilib>:"Start.vi"("error in (no error)"=w332, "SMO"=w336) -> ("error out"=w331:errorcluster, "SMO out"=w333:refnum<class "ExampleInstrument.lvclass">)  [unwired: 8 in]
        n118 = Bundle By Name(cluster=w335, "Instrument"=w333) -> (w334:T4)
        n119 = call <vilib>:"Add State(s) to Queue__jki_lib_state_machine.vi"("State(s) in (\"\")"=w339) -> ("States Out"=w338:string)  [unwired: 14 in]
      }
      frame "SMO: Create Instrument UI" {
        # "Do not put any code in this frame.\n(It is a separator no-op. You can make a copy of this frame to create a new Macro frame)"
        n120 = Unbundle By Name(w346) -> ("Instrument UI"=w344:refnum<class "ExampleInstrument.UI.lvclass">, "Instrument"=w343:refnum<class "ExampleInstrument.lvclass">)
        n121 = call "ExampleInstrument.UI.Create UI.vi"("error in (no error)"=w341, "Instrument in"=w343, "Example Instrument UI in"=w344) -> ("error out"=w340:errorcluster, "Example Instrument UI out"=w342:refnum<class "ExampleInstrument.UI.lvclass">)  [unwired: 7 in]
        n122 = Bundle By Name(cluster=w346, "Instrument UI"=w342) -> (w345:T4)
        n123 = call <vilib>:"Add State(s) to Queue__jki_lib_state_machine.vi"("State(s) in (\"\")"=w349) -> ("States Out"=w348:string)  [unwired: 14 in]
      }
      frame "SMO: Start Instrument UI" {
        # "Do not put any code in this frame.\n(It is a separator no-op. You can make a copy of this frame to create a new Macro frame)"
        n124 = Unbundle By Name(w353) -> ("Instrument UI"=w352:refnum<class "ExampleInstrument.UI.lvclass">)
        n125 = call <vilib>:"Start.vi"("error in (no error)"=w351, "SMO"=w352) -> ("error out"=w350:errorcluster)  [unwired: 8 in, 1 out]
        n126 = call <vilib>:"Add State(s) to Queue__jki_lib_state_machine.vi"("State(s) in (\"\")"=w356) -> ("States Out"=w355:string)  [unwired: 14 in]
      }
      frame "SMO: Show Instrument UI" {
        # "Do not put any code in this frame.\n(It is a separator no-op. You can make a copy of this frame to create a new Macro frame)"
        n127 = Unbundle By Name(w364) -> ("Instrument UI"=w362:refnum<class "ExampleInstrument.UI.lvclass">)
        n128 = call <vilib>:"GetState.vi"("error in (no error)"=w360, "SMO"=w362) -> ("error out"=w358:errorcluster, "SMO State"=w357:T1, "SMO out"=w361:refnum<class "ExampleInstrument.UI.lvclass">)  [unwired: 7 in]
        n129 = call <vilib>:"Clear Errors.vi"("error in (no error)"=w358) -> ("error out"=w359:errorcluster)  [unwired: 5 in, 1 out]
        n130 = case shown="Default" w357 {
          tunnel: [w368 w371] -> w363
          tunnel: w361 -> [_ w370]
          tunnel: w359 -> [w368 w369]
          frame Default {
          }
          frame "Started" {
            n131 = call <vilib>:"Show.vi"("error in (no error)"=w369, "SMO.UI"=w370) -> ("error out"=w371:errorcluster)  [unwired: 8 in, 1 out]
          }
        }
        n132 = call <vilib>:"Add State(s) to Queue__jki_lib_state_machine.vi"("State(s) in (\"\")"=w367) -> ("States Out"=w366:string)  [unwired: 14 in]
      }
      frame "SMO: Destroy Instrument" {
        # "Do not put any code in this frame.\n(It is a separator no-op. You can make a copy of this frame to create a new Macro frame)"
        n133 = Unbundle By Name(w379) -> ("Instrument"=w377:refnum<class "ExampleInstrument.lvclass">)
        n134 = call <vilib>:"GetState.vi"("error in (no error)"=w374, "SMO"=w377) -> ("error out"=w373:errorcluster, "SMO State"=w376:T1, "SMO out"=w372:refnum<class "ExampleInstrument.lvclass">)  [unwired: 7 in]
        n135 = call <vilib>:"Clear Errors.vi"("error in (no error)"=w373) -> ("error out"=w375:errorcluster)  [unwired: 5 in, 1 out]
        n136 = case shown="Default" w376 {
          tunnel: [w383 w386] -> w378
          tunnel: w375 -> [w383 w385]
          tunnel: w372 -> [_ w384]
          frame Default {
          }
          frame "Stopped" {
            n137 = call <vilib>:"Destroy.vi"("error in (no error)"=w385, "SMO"=w384) -> ("error out"=w386:errorcluster)  [unwired: 9 in]
          }
        }
        n138 = call <vilib>:"Add State(s) to Queue__jki_lib_state_machine.vi"("State(s) in (\"\")"=w382) -> ("States Out"=w381:string)  [unwired: 14 in]
      }
      frame "SMO: Hide Instrument UI" {
        # "Do not put any code in this frame.\n(It is a separator no-op. You can make a copy of this frame to create a new Macro frame)"
        n139 = Unbundle By Name(w394) -> ("Instrument UI"=w392:refnum<class "ExampleInstrument.UI.lvclass">)
        n140 = call <vilib>:"GetState.vi"("error in (no error)"=w390, "SMO"=w392) -> ("error out"=w388:errorcluster, "SMO State"=w387:T1, "SMO out"=w391:refnum<class "ExampleInstrument.UI.lvclass">)  [unwired: 7 in]
        n141 = call <vilib>:"Clear Errors.vi"("error in (no error)"=w388) -> ("error out"=w389:errorcluster)  [unwired: 5 in, 1 out]
        n142 = case shown="Default" w387 {
          tunnel: [w398 w401] -> w393
          tunnel: w391 -> [_ w400]
          tunnel: w389 -> [w398 w399]
          frame Default {
          }
          frame "Started" {
            n143 = call <vilib>:"Hide.vi"("error in (no error)"=w399, "SMO.UI"=w400) -> ("error out"=w401:errorcluster)  [unwired: 8 in, 1 out]
          }
        }
        n144 = call <vilib>:"Add State(s) to Queue__jki_lib_state_machine.vi"("State(s) in (\"\")"=w397) -> ("States Out"=w396:string)  [unwired: 14 in]
      }
      frame "SMO: Stop Instrument UI" {
        # "Do not put any code in this frame.\n(It is a separator no-op. You can make a copy of this frame to create a new Macro frame)"
        n145 = Unbundle By Name(w408) -> ("Instrument UI"=w403:refnum<class "ExampleInstrument.UI.lvclass">)
        n146 = call <vilib>:"GetState.vi"("error in (no error)"=w407, "SMO"=w403) -> ("error out"=w406:errorcluster, "SMO State"=w404:T1, "SMO out"=w402:refnum<class "ExampleInstrument.UI.lvclass">)  [unwired: 7 in]
        n147 = call <vilib>:"Clear Errors.vi"("error in (no error)"=w406) -> ("error out"=w405:errorcluster)  [unwired: 5 in, 1 out]
        n148 = case shown="\"Created\", \"Started\"" w404 {
          tunnel: [w413 w416] -> w409
          tunnel: w402 -> [_ w415]
          tunnel: w405 -> [w413 w414]
          frame Default {
          }
          frame "Created", "Started" {
            n149 = call <vilib>:"Stop.vi"("error in (no error)"=w414, "SMO"=w415) -> ("error out"=w416:errorcluster)  [unwired: 8 in, 1 out]
          }
        }
        n150 = call <vilib>:"Add State(s) to Queue__jki_lib_state_machine.vi"("State(s) in (\"\")"=w412) -> ("States Out"=w411:string)  [unwired: 14 in]
      }
      frame "SMO: Destroy Instrument UI" {
        # "Do not put any code in this frame.\n(It is a separator no-op. You can make a copy of this frame to create a new Macro frame)"
        n151 = Unbundle By Name(w423) -> ("Instrument UI"=w422:refnum<class "ExampleInstrument.UI.lvclass">)
        n152 = call <vilib>:"GetState.vi"("error in (no error)"=w420, "SMO"=w422) -> ("error out"=w419:errorcluster, "SMO State"=w417:T1, "SMO out"=w421:refnum<class "ExampleInstrument.UI.lvclass">)  [unwired: 7 in]
        n153 = call <vilib>:"Clear Errors.vi"("error in (no error)"=w419) -> ("error out"=w418:errorcluster)  [unwired: 5 in, 1 out]
        n154 = case shown="Default" w417 {
          tunnel: w418 -> [w428 w431]
          tunnel: [w428 w430] -> w424
          tunnel: w421 -> [_ w429]
          frame Default {
          }
          frame "Stopped" {
            n155 = call <vilib>:"Destroy.vi"("error in (no error)"=w431, "SMO"=w429) -> ("error out"=w430:errorcluster)  [unwired: 9 in]
          }
        }
        n156 = call <vilib>:"Add State(s) to Queue__jki_lib_state_machine.vi"("State(s) in (\"\")"=w427) -> ("States Out"=w426:string)  [unwired: 14 in]
      }
      frame "---------- Splash ----------" {
        # "Template Separator\n(You can make a copy of, or modify, this frame)"
        n157 = call <vilib>:"Add State(s) to Queue__jki_lib_state_machine.vi"("State(s) in (\"\")"=w436) -> ("States Out"=w435:string)  [unwired: 14 in]
      }
      frame "Splash: Set Status" {
        # "Your code here.\n(You can make a copy of, or modify, this frame)"
        n158 = property on="Splash Status" class="Str"(error in=w439, "Value"=w440) -> (error out=w438:errorcluster)  [unwired: 1 in, 1 out]
        n159 = call <vilib>:"Add State(s) to Queue__jki_lib_state_machine.vi"("State(s) in (\"\")"=w443) -> ("States Out"=w442:string)  [unwired: 14 in]
      }
      frame "Splash: 2" {
        # "Your code here.\n(You can make a copy of, or modify, this frame)"
        n160 = call <vilib>:"Add State(s) to Queue__jki_lib_state_machine.vi"("State(s) in (\"\")"=w448) -> ("States Out"=w447:string)  [unwired: 14 in]
      }
    }
  }
  "error out" <- w1
